vi "LVClass_HasoSlopes Apply Substractor.vi"(0 "HasoSlopes in":refnum<class "HasoSlopes.lvclass">, 7 "HasoSlopes to substract":refnum<class "HasoSlopes.lvclass">, 11 "error in (no error)":errorcluster) -> (4 "HasoSlopes out":refnum<class "HasoSlopes.lvclass">, 15 "error out":errorcluster)   [LabVIEW 2020, in "HasoSlopes.lvclass"]
uses:
  HasoSlopes.lvclass
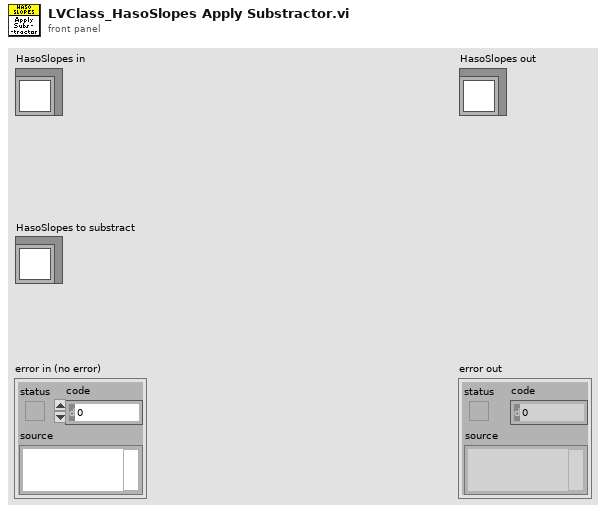
[diagram p1: front panel]
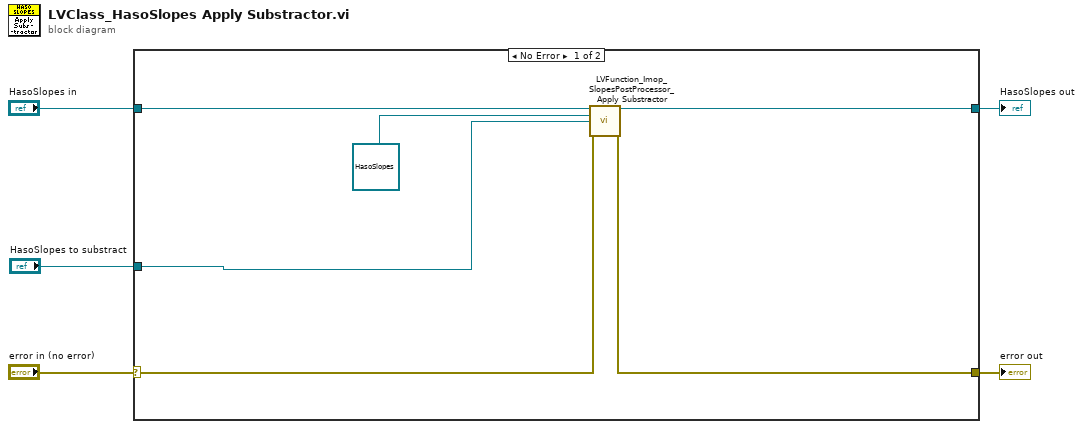
[diagram p0: block diagram]
diagram:
  n1 = case shown="No Error" "error in (no error)" {
    selector: "error in (no error)" -> [w8 w13]
    tunnel: [w7 w13] -> w4
    tunnel: [w10 w12] -> w2
    tunnel: "HasoSlopes in" -> [w11 w12]
    tunnel: "HasoSlopes to substract" -> [w9 _]
    frame No Error {
      n2 = call "LVFunction_Imop_SlopesPostProcessor_Apply Substractor.vi"("HasoSlopes in"=w11, "HasoSlopes OUT"=refnum<class "HasoSlopes.lvclass"> refnum, "HasoSlopes to substract"=w9, "error in (no error)"=w8) -> ("HasoSlopes out"=w10:refnum<class "HasoSlopes.lvclass">, "error out"=w7:errorcluster)  [unwired: 9 in, 1 out]
    }
    frame Error {
    }
  }
  "error out" <- w4
  "HasoSlopes out" <- w2
